vi "PCert-ConfigPageNF-Initialize.vi"(9 "FTW Actor Instance Configuration":string="{\n  \"Identity\": \"ActorName\",\n  \"InboxAddress\": \"tcp://127.0.0.1:*\",\n  \"PublisherAddress\": \"tcp://127.0.0.1:*\",\n  \"DebugEnableInboxLogging\": false,\n  \"DebugEnableJobLogging\": false,\n  \"DebugShowPanel\": false\n}", 10 "Initialization Job Sequence":string, 11 "ERP-ConfigPageNF.lvclass":refnum<class "PCert-ConfigPageNF.lvclass">) -> (0 "error out":errorcluster, 3 "ERP-ConfigPageNF out":refnum<class "PCert-ConfigPageNF.lvclass">)   [LabVIEW 2013, in "PCert-ConfigPageNF.lvclass"]
uses:
  PCert-ConfigPageNF.lvclass
  PCert-ConfigPageNF.lvclass/PCert-ConfigPageNF.ctl
  ftw-dataflow/Actor/src/Connector/FTW-ActorConnector.lvclass
  ftw-dataflow/Core/src/Reflection/FTW-Reflection-Type.vi
  ftw-dataflow/Core/src/JSON/FTW-JSON-Core-LibraryFilepath.vi
  ftw-dataflow/Core/src/JSON/FTW-JSON-Core-GetFlattenedValue.vi
  ftw-dataflow/Core/src/JSON/FTW-JSON-Core-LibraryError.vi
  ftw-dataflow/Core/utils/CodeGen/JSON Deserialize/FTW-JSON-Deserialize.xnode
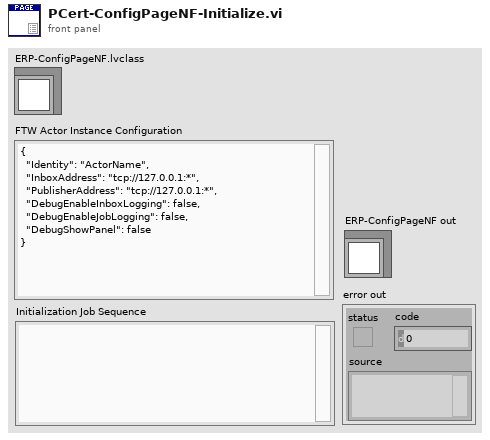
[diagram p1: front panel]
types:
  T1 = cluster{"ContainerAddress":string, "DatabaseAddress":string}
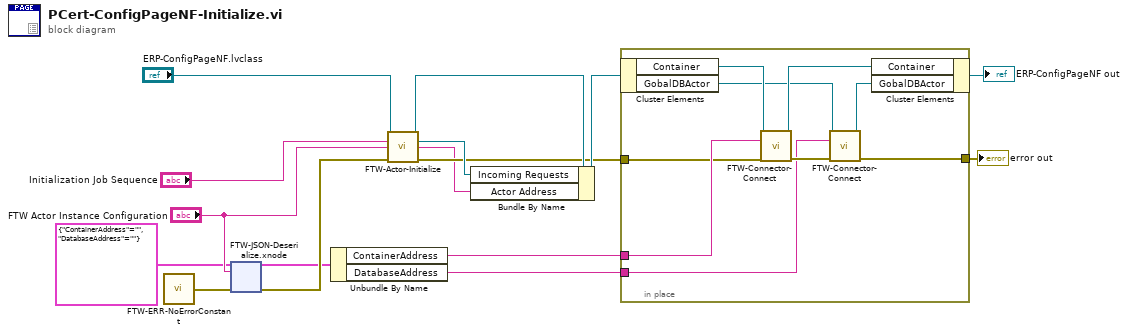
[diagram p0: block diagram]
diagram:
  n1 = call "FTW-ERR-NoErrorConstant.vi"() -> ("no error"=w14:errorcluster)
  n2 = xnode "FTW-JSON-Deserialize.xnode"("Type and Defaults"=T1 {"ContainerAddress"="", "DatabaseAddress"=""}, "JSON String"="FTW Actor Instance Configuration", "error in"=w14) -> ("Values"=w1:T1, "error out"=w13:errorcluster)
  n3 = Unbundle By Name(w1) -> ("ContainerAddress"=w9:string, "DatabaseAddress"=w4:string)
  n4 = call-dynamic "FTW-Actor-Initialize.vi"("FTW Actor Instance Type"="ERP-ConfigPageNF.lvclass", "Initialization Job Sequence"="Initialization Job Sequence", "Actor Instance Configuration"="FTW Actor Instance Configuration", "error in"=w13) -> ("FTW Actor Instance"=w11:refnum<class "PCert-ConfigPageNF.lvclass">, "Incoming Requests"=w12:refnum<event-registration>, "Actual Server Address"=w5:string, "error out"=w8:errorcluster)  [unwired: 8 in]
  n5 = Bundle By Name(cluster=w11, "Incoming Requests"=w12, "Actor Address"=w5) -> (w10:refnum<class "PCert-ConfigPageNF.lvclass">)
  n6 = in-place {
    in-place-border: w9 -> [w24]
    in-place-border: w8 -> [w23]
    in-place-border: [w17] -> w6
    in-place-border: w4 -> [w19]
    n7 = in-place-cluster #1(w10) -> ("Container"=w25:refnum<class "FTW-ActorConnector.lvclass">, "GobalDBActor"=w21:refnum<class "FTW-ActorConnector.lvclass">)
    n8 = call-dynamic "FTW-Connector-Connect.vi"("FTW Actor Connector Type"=w25, "Instance Inbox Address"=w24, "error in"=w23) -> ("FTW Actor Connector"=w22:refnum<class "FTW-ActorConnector.lvclass">, "error out"=w20:errorcluster)  [unwired: 11 in]
    n9 = call-dynamic "FTW-Connector-Connect.vi"("FTW Actor Connector Type"=w21, "Instance Inbox Address"=w19, "error in"=w20) -> ("FTW Actor Connector"=w18:refnum<class "FTW-ActorConnector.lvclass">, "error out"=w17:errorcluster)  [unwired: 11 in]
    n10 = in-place-cluster #1("Container"=w22, "GobalDBActor"=w18) -> (→"ERP-ConfigPageNF out":refnum<class "PCert-ConfigPageNF.lvclass">)
  }
  "error out" <- w6
